vi "Rej_szybka_obwiednia_old.vi"(6 "Liczba probek (200)":i32(slide)=200 min=0 max=400 step=20 scale=0.0..400.0, 8 "error in (no error)":errorcluster, 11 "Wfm in":waveform(dbl)) -> (0 "error out":errorcluster, 2 "Wfm min out":waveform(dbl), 3 "Wfm max out":waveform(dbl))   [LabVIEW 2013]
doc: "Liczy obwiednie (gorna -> max i dolna -> min) sygnalu\nLiczba probek zadawana"
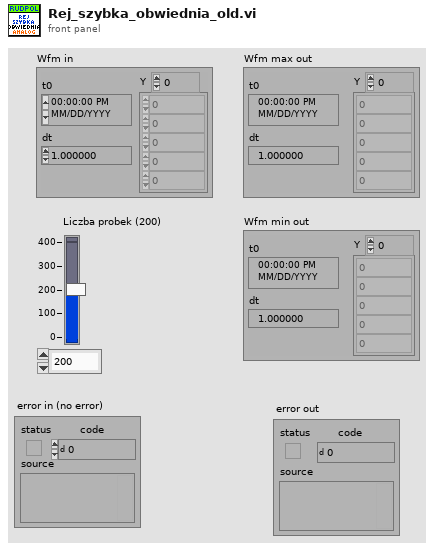
[diagram p1: front panel]
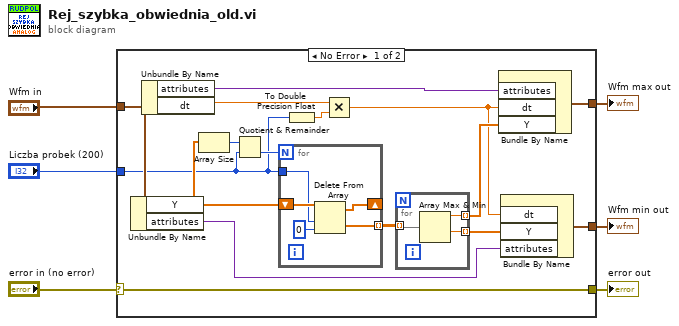
[diagram p0: block diagram]
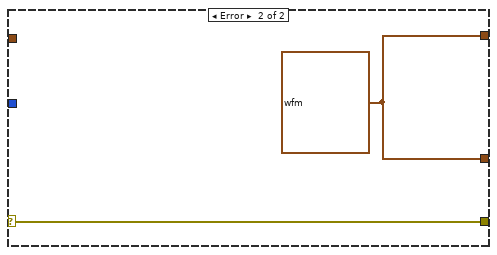
[diagram p2: hidden frame]
diagram:
  n1 = case shown="No Error" "error in (no error)" {
    selector: "error in (no error)" -> [w22 w32]
    tunnel: [w22 w32] -> w6
    tunnel: [w12 w31] -> w4
    tunnel: [w11 w31] -> w3
    tunnel: "Wfm in" -> [w10 _]
    tunnel: "Liczba probek (200)" -> [w9 _]
    frame No Error {
      n2 = Unbundle By Name(w10) -> ("Y"=w21:dbl[], "attributes"=w8:variant)
      n3 = Unbundle By Name(w10) -> ("attributes"=w7:variant, "dt"=w19:dbl)
      n4 = Array Size(array=w21) -> (size(s)=w15:i32)
      n5 = Quotient & Remainder(x=w15, y=w9) -> (floor(x/y)=w14:i32)  [unwired: 1 out]
      n6 = for {
        N: w14 -> [_]
        shift-right: [w29] -> _
        shift-left: w21 -> [w30]
        tunnel: [w28] -> w20 mode=indexing
        tunnel: w9 -> [w27]
        n7 = Delete From Array(array=w30, length=w27, index=0) -> (deleted portion=w28:dbl[], array with subset deleted=w29:dbl[])
      }
      n8 = To Double Precision Float(number=w9) -> (double precision float=w13:dbl)
      n9 = Multiply(x=w19, y=w13) -> (x*y=w16:dbl)
      n10 = for {
        tunnel: w20 -> [w25] mode=indexing
        tunnel: [w24] -> w18 mode=indexing
        tunnel: [w23] -> w17 mode=indexing
        n11 = Array Max & Min(array=w25) -> (max value=w24:dbl, min value=w23:dbl)  [unwired: 2 out]
      }
      n12 = Bundle By Name("attributes"=w7, "dt"=w16, "Y"=w18) -> (w11:waveform(dbl))  [unwired: 1 in]
      n13 = Bundle By Name("dt"=w16, "Y"=w17, "attributes"=w8) -> (w12:waveform(dbl))  [unwired: 1 in]
    }
    frame Error {
      w31 = waveform(dbl) {"t0"=timestamp(0 s since 1904-01-01), "dt"=1.0, "Y"=[]}
    }
  }
  "Wfm max out" <- w3
  "Wfm min out" <- w4
  "error out" <- w6
